vi "读取VISA Resource.vi"(8 "error in (no error)":errorcluster caption="错误输入（无错误）", 11 "HL7输入":refnum<class "HL7.lvclass">) -> (0 "error out":errorcluster caption="错误输出", 2 "VISA Resource":refnum<visa-resource-name>, 3 "HL7输出":refnum<class "HL7.lvclass">)   [LabVIEW 2016, in "HL7.lvlib" / "HL7.lvclass"]
uses:
  HL7.lvclass
  HL7.lvclass/HL7.ctl
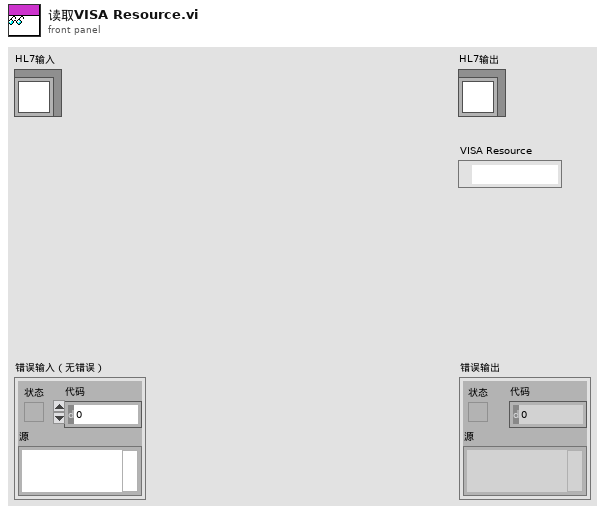
[diagram p1: front panel]
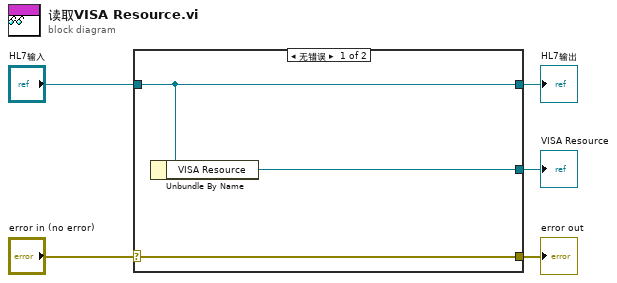
[diagram p0: block diagram]
diagram:
  n1 = case shown="无错误" "error in (no error)" {
    selector: "error in (no error)" -> [w8 w9]
    tunnel: [w8 w9] -> w4
    tunnel: [w7 w10] -> w2
    tunnel: "HL7输入" -> [w7 w10]
    tunnel: [w6 _] -> w1
    frame No Error {
      n2 = Unbundle By Name(w7) -> ("VISA Resource"=w6:refnum<visa-resource-name>)
    }
    frame Error {
    }
  }
  "error out" <- w4
  "HL7输出" <- w2
  "VISA Resource" <- w1
